vi "ReadFilesOnes.vi"(11 "prompt":string) -> (1 "number of bytes":i64, 2 "Size":i32, 3 "Data":u8[](array[numeric]))   [LabVIEW 2015]
panel:
  in  "#ofData":i32=10
  in  "IndexNextSection":i64
  out "IndexNextSection":dbl
  in  "m":dbl=2.0
  in  "#ofSections":u8=1
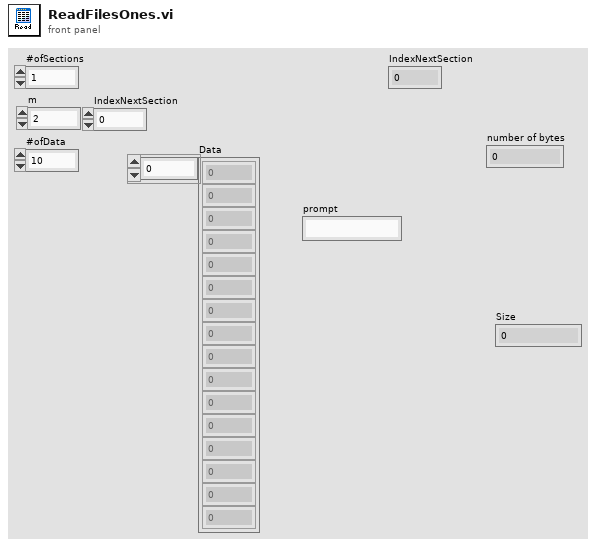
[diagram p1: front panel]
types:
  T1 = enum16{"big-endian, network order", "native, host order", "little-endian"}
  T2 = enum16{"open", "replace", "create", "open or create", "replace or create", "replace or create with confirmation"}
  T3 = enum16{"deny read/write", "deny write-only", "deny none"}
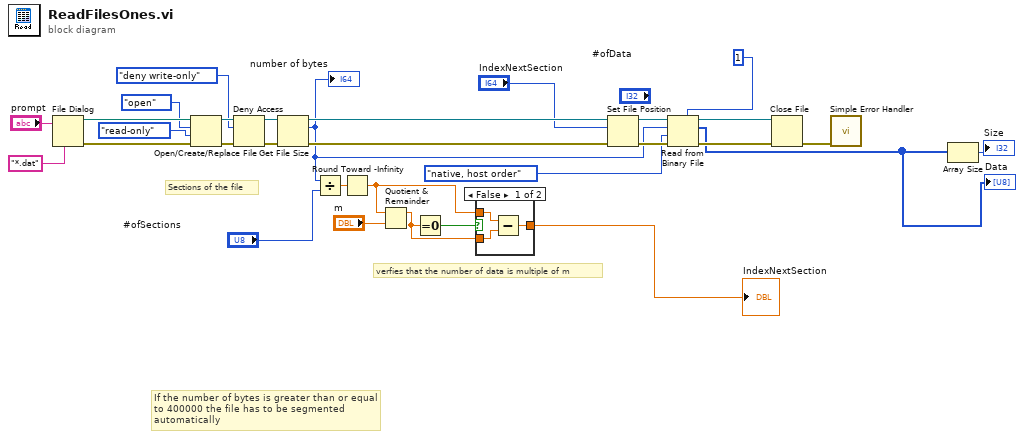
[diagram p0: block diagram]
diagram:
  # "verfies that the number of data is multiple of m"
  # "Sections of the file"
  # "If the number of bytes is greater than or equal\nto 400000 the file has to be segmented\nautomatically"
  n1 = File Dialog(6:"*.dat" ("pattern (all files)"), 7:"prompt") -> (0:w29:errorcluster, 3:w31:path)  [unwired: 5 in, 2 out]
  n2 = Open/Create/Replace File(file path (use dialog)=w31, error in=w29, operation (0:open)=T2."open", access (0:read/write)=enum16{"read/write", "read-only", "write-only"}."read-only") -> (refnum out=w26:refnum<file>, error out=w27:errorcluster)  [unwired: 2 in, 1 out]
  n3 = Deny Access(4:w27, 6:T3."deny write-only" ("deny mode (0:deny read/write)"), 7:w26) -> (0:w25:errorcluster, 3:w22:refnum<file>)
  n4 = Get File Size(file=w22, error in=w25) -> (refnum out=w21:refnum<file>, size (in bytes)=w3:i64, 0:w20:errorcluster)
  "number of bytes" <- w3
  n5 = Divide(x=w3, y="#ofSections") -> (x/y=w9:dbl)
  n6 = Round Toward -Infinity(1:w9) -> (0:w8:dbl)
  n7 = Quotient & Remainder(x=w8, y="m") -> (x-y*floor(x/y)=w10:dbl)  [unwired: 1 out]
  n8 = Equal To 0?(x=w10) -> (x = 0?=w11:bool)
  n9 = case shown="False" w11 {
    tunnel: [w32 w35] -> w4
    tunnel: w8 -> [w34 w35]
    tunnel: w10 -> [w33 _]
    frame False {
      n10 = Subtract(x=w34, y=w33) -> (x-y=w32:dbl)
    }
    frame True {
    }
  }
  "IndexNextSection" <- w4
  n11 = Set File Position(offset (in bytes) (0)="IndexNextSection", refnum=w21, error in=w20) -> (refnum out=w16:refnum<file>, error out=w15:errorcluster)  [unwired: 1 in]
  n12 = Read from Binary File(5:u8 1 ("Data Type (DBL)"), 8:w15, 9:T1."native, host order" ("byte order (0:big-endian, network order)"), 10:w3, 11:w16) -> (0:w17:errorcluster, 2:w1:u8[], 3:w18:refnum<file>)  [unwired: 1 in, 1 out]
  "Data" <- w1
  n13 = Close File(refnum=w18, error in=w17) -> (error out=w19:errorcluster)  [unwired: 1 out]
  n14 = call <vilib>:"Simple Error Handler.vi"("error in (no error)"=w19) -> ()  [unwired: 4 in, 5 out]
  n15 = Array Size(array=w1) -> (size(s)=→"Size":i32)
